vi "SetJogAcceleration.vi"(8 "error in (no error)":errorcluster, 10 "Jog Acceleration":dbl, 11 "ThorlabsLabJack in":refnum<class "ThorlabsLabJack.lvclass">) -> (0 "error out":errorcluster, 3 "ThorlabsLabJack out":refnum<class "ThorlabsLabJack.lvclass">)   [LabVIEW 2018, in "ThorlabsLabJack.lvlib" / "ThorlabsLabJack.lvclass"]
uses:
  ThorlabsLabJack.lvclass
  ThorlabsLabJack.lvclass/ThorlabsLabJack.ctl
  C:/Projects/LabVIEW/In-Progress/Chetan Malpure/Axis/Thorlabs LabJack/Drivers/Thorlabs.MotionControl.IntegratedStepperMotorsCLI.dll
  Drivers/Thorlabs.MotionControl.IntegratedStepperMotorsCLI.dll
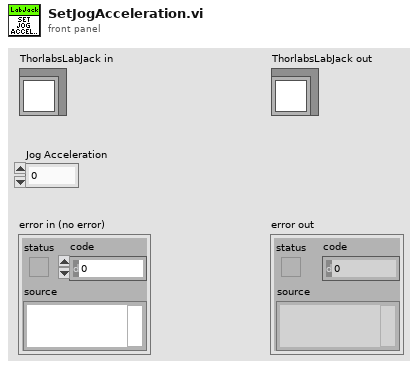
[diagram p1: front panel]
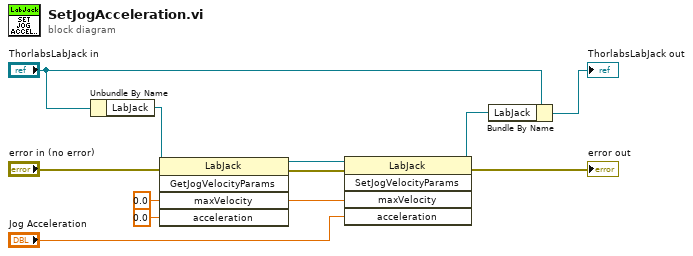
[diagram p0: block diagram]
diagram:
  n1 = Unbundle By Name("ThorlabsLabJack in") -> ("LabJack"=w8:refnum<k24>)
  n2 = invoke class="LabJack" method="GetJogVelocityParams"(reference=w8, error in="error in (no error)", "maxVelocity"=0.0, "acceleration"=0.0) -> (reference out=w5:refnum<k24>, error out=w6:errorcluster, "maxVelocity"=w1:dbl)  [unwired: 1 in, 2 out]
  n3 = invoke class="LabJack" method="SetJogVelocityParams"(reference=w5, error in=w6, "maxVelocity"=w1, "acceleration"="Jog Acceleration") -> (reference out=w9:refnum<k24>, error out=→"error out":errorcluster)  [unwired: 1 in, 3 out]
  n4 = Bundle By Name(cluster="ThorlabsLabJack in", "LabJack"=w9) -> (→"ThorlabsLabJack out":refnum<class "ThorlabsLabJack.lvclass">)
